vi "Write DAQ Parameters.vi"(8 "error in (no error)":errorcluster, 10 "DAQ Parameters":T1, 11 "ATS9462 Class in":refnum<class "ATS9462 Class.lvclass">) -> (0 "error out":errorcluster, 3 "ATS9462 Class out":refnum<class "ATS9462 Class.lvclass">)   [LabVIEW 2014, in "ATS9462 Class.lvclass"]
uses:
  ATS9462 Class.lvclass
  DAQ Parameters.ctl
  Trigger Source.ctl
  Trigger Slope.ctl
  Type Defs/OCT DAQ Channel Data Type.ctl
  Clock Control.ctl
  ATS-VI/ATS_ctl/ATS_Global.ctl
  ATS-VI/ATS_ctl/Record.ctl
  ATS-VI/ATS_ctl/Clock.ctl
  ATS-VI/ATS_ctl/ClockSource.ctl
  ATS-VI/ATS_ctl/ClockRate.ctl
  ATS-VI/ATS_ctl/ClockEdge.ctl
  ATS-VI/ATS_ctl/InputCtrl.ctl
  ATS-VI/ATS_ctl/Coupling.ctl
  ATS-VI/ATS_ctl/Range.ctl
  ATS-VI/ATS_ctl/Impedance.ctl
  ATS-VI/ATS_ctl/Bandwidth.ctl
  ATS-VI/ATS_ctl/Trigger.ctl
  ATS-VI/ATS_ctl/TriggerOperation.ctl
  ATS-VI/ATS_ctl/TriggerEngine.ctl
  ATS-VI/ATS_ctl/ExtTrigger.ctl
  ATS-VI/ATS_ctl/ExtTrigRange.ctl
  ATS-VI/ATS_ctl/ATS_Async_Ctrl.ctl
  ATS-VI/ATS_ctl/ATS_Async_Mode.ctl
  ATS-VI/ATS_ctl/ATS_ReadSamples.ctl
  ATS-VI/ATS_ctl/ATS_Async_Setting.ctl
  ATS9462 Class.lvclass/ATS9462 Class.ctl
  ATS-VI/ATS_ctl/ATS_DMA_Channel.ctl
  DAQ Class.lvclass
panel:
  out "Return Code":u32
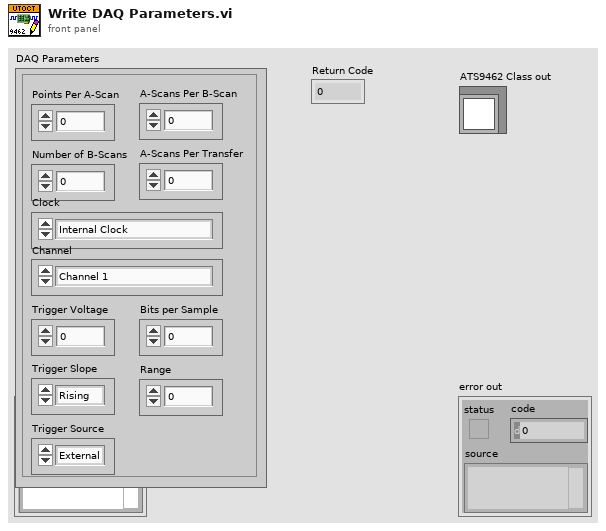
[diagram p1: front panel]
types:
  T1 = typedef "DAQ Class.lvclass/DAQ Parameters.ctl" = cluster{"Points Per A-Scan":u32, "A-Scans Per B-Scan":u32, "Number of B-Scans":u32, "A-Scans Per Transfer":u32, "Trigger Voltage":sgl, "Trigger Source":T2, "Trigger Slope":T3, "Channel":T4, "Clock":T5, "Bits per Sample":dbl, "Range":dbl}
  T2 = typedef "DAQ Class.lvclass/Trigger Source.ctl" = enum16{"External", "Channel A", "Channel B"}
  T3 = typedef "DAQ Class.lvclass/Trigger Slope.ctl" = enum16{"Rising", "Falling"}
  T4 = typedef "OCT DAQ Channel Data Type.ctl" = enum16{"Channel 1", "Channel 2", "Channel 1 and 2"}
  T5 = typedef "DAQ Class.lvclass/Clock Control.ctl" = enum16{"Internal Clock", "External Clock"}
  T6 = typedef "ClockRate.ctl" = u32
  T7 = typedef "ATS_Async_Setting.ctl" = cluster{"UseHeader":u32, "Rec/Buffer":u32, "Total_Rec":u32, "DataBuffer":bool, "GetProcessedData":bool}
  T8 = typedef "ATS_ReadSamples.ctl" = cluster{"Offset":i32, "Length":u32}
  T9 = typedef "ATS_Async_Mode.ctl" = enum16{"Continuous", "Triggered", "No-Pre-Trigger", "Traditional"}
  T10 = typedef "ATS_Async_Ctrl.ctl" = enum16{"SetupDMA", "StartCapture", "Get", "Get_Stream", "Abort", "Stop"}
  T11 = typedef "ATS_Global.ctl" = cluster{"Record":T12, "Clock":T13, "Input A":T16, "Input B":T16, "Trigger":T21}
  T12 = typedef "Record.ctl" = cluster{"Count":u32, "Presize":u32, "Length":u32}
  T13 = typedef "Clock.ctl" = cluster{"ClckSource":T14, "ClckRate":T6, "ClckEdge":T15, "Decimation":u32}
  T14 = typedef "ClockSource.ctl" = enum16{"Internal", "External", "Medium Ext.", "Slow Ext.", "Ext. AC", "Ext. DC", "Ext. (PLL)"}
  T15 = typedef "ClockEdge.ctl" = u16
  T16 = typedef "InputCtrl.ctl" = cluster{"Coupling":T17, "Range":T18, "Impedance":T19, "Bandwidth":T20}
  T17 = typedef "Coupling.ctl" = enum16{"AC", "DC"}
  T18 = typedef "Range.ctl" = u32
  T19 = typedef "Impedance.ctl" = enum16{"1M ohms", "50 ohms"}
  T20 = typedef "Bandwidth.ctl" = enum16{"Full Bandwidth", "Reduce Bandwidth"}
  T21 = typedef "Trigger.ctl" = cluster{"TrigOperation":T22, "Timeout (s)":dbl, "Trig. Delay":u32, "Engine X":T23, "Engine Y":T23, "ExtTrigControl":T24}
  T22 = typedef "TriggerOperation.ctl" = enum16{"Only X", "Only Y", "X or Y", "X and Y", "X xor Y", "X and not Y", "not X and Y"}
  T23 = typedef "TriggerEngine.ctl" = cluster{"Source":enum32{"Chan_A", "Chan_B", "External", "Disable"}, "Slope":enum32{"Positive", "Negative"}, "Level":u32}
  T24 = typedef "ExtTrigger.ctl" = cluster{"Coupling":T17, "Range":T25}
  T25 = typedef "ExtTrigRange.ctl" = enum16{"1 V", "5 V", "TTL"}
  T26 = enum32{"Chan_A", "Chan_B", "External", "Disable"}
  T27 = typedef "ATS_DMA_Channel.ctl" = enum16{"Channel_A", "Channel_B", "A & B"}
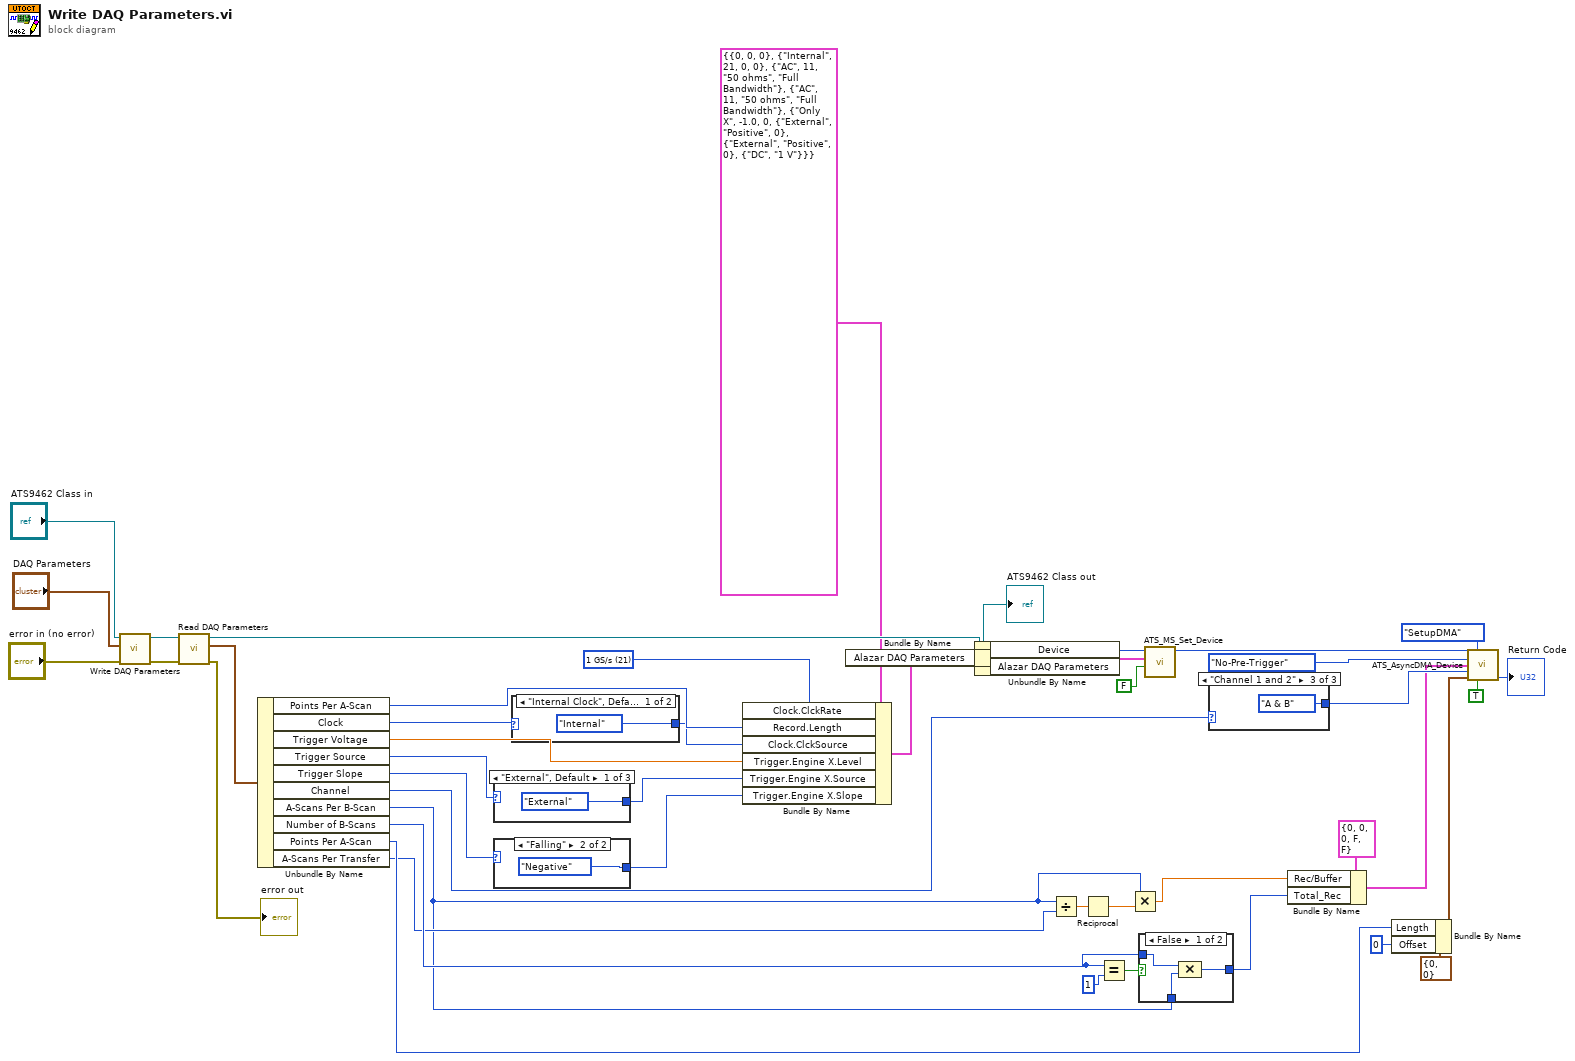
[diagram p0: block diagram]
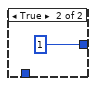
[diagram p2: hidden frame]
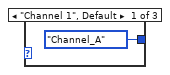
[diagram p3: hidden frame]
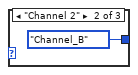
[diagram p4: hidden frame]
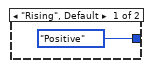
[diagram p5: hidden frame]
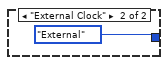
[diagram p6: hidden frame]
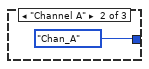
[diagram p7: hidden frame]
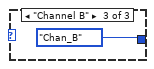
[diagram p8: hidden frame]
diagram:
  w11 = T6 21 items=["1 kS/s", "2 kS/s", "5 kS/s", "10 kS/s", "20 kS/s", "50 kS/s", "100 kS/s", "200 kS/s", "500 kS/s", "1 MS/s", "2 MS/s", "5 MS/s", "10 MS/s", "20 MS/s", "25 MS/s", "50 MS/s", "100 MS/s", "125 MS/s", "200 MS/s", "250 MS/s", "500 MS/s", "1 GS/s"] ("Clock.ClckRate")
  n1 = call-parent "Write DAQ Parameters.vi"("error in (no error)"="error in (no error)", "DAQ Parameters"="DAQ Parameters", "DAQ Class in"="ATS9462 Class in") -> ("error out"=w41:errorcluster, "DAQ Class out"=w42:refnum<class "ATS9462 Class.lvclass">)  [unwired: 7 in]
  n2 = call-dynamic "Read DAQ Parameters.vi"("error in (no error)"=w41, "ATS9462 Class in"=w42) -> ("error out"=→"error out":errorcluster, "DAQ Parameters"=w40:T1, "ATS9462 Class out"=w33:refnum<class "ATS9462 Class.lvclass">)  [unwired: 7 in]
  n3 = Unbundle By Name(w40) -> ("Points Per A-Scan"=w37:u32, "Clock"=w36:T5, "Trigger Voltage"=w34:sgl, "Trigger Source"=w39:T2, "Trigger Slope"=w32:T3, "Channel"=w24:T4, "A-Scans Per B-Scan"=w1:u32, "Number of B-Scans"=w7:u32, "Points Per A-Scan"=w13:u32, "A-Scans Per Transfer"=w2:u32)
  n4 = case shown="\"External\", Default" w39 {
    tunnel: [T26."External" ("Trigger.Engine X.Source") T26."Chan_A" ("Trigger.Engine X.Source") T26."Chan_B" ("Trigger.Engine X.Source")] -> w38
    frame "External", Default {
    }
    frame "Channel A" {
    }
    frame "Channel B" {
    }
  }
  n5 = case shown="\"Falling\"" w32 {
    tunnel: [enum32{"Positive", "Negative"}."Positive" ("Trigger.Engine X.Slope") enum32{"Positive", "Negative"}."Negative" ("Trigger.Engine X.Slope")] -> w31
    frame "Rising", Default {
    }
    frame "Falling" {
    }
  }
  n6 = case shown="\"Internal Clock\", Default" w36 {
    tunnel: [ClockSource."Internal" ("Clock.ClckSource") ClockSource."External" ("Clock.ClckSource")] -> w35
    frame "Internal Clock", Default {
    }
    frame "External Clock" {
    }
  }
  n7 = Bundle By Name(cluster=T11 {"Record"={"Count"=0, "Presize"=0, "Length"=0}, "Clock"={"ClckSource"=enum."Internal", "ClckRate"=21, "ClckEdge"=0, "Decimation"=0}, "Input A"={"Coupling"=enum."AC", "Range"=11, "Impedance"=enum."50 ohms", "Bandwidth"=enum."Full Bandwidth"}, "Input B"={"Coupling"=enum."AC", "Range"=11, "Impedance"=enum."50 ohms", "Bandwidth"=enum."Full Bandwidth"}, "Trigger"={"TrigOperation"=enum."Only X", "Timeout (s)"=-1.0, "Trig. Delay"=0, "Engine X"={"Source"=enum."External", "Slope"=enum."Positive", "Level"=0}, "Engine Y"={"Source"=enum."External", "Slope"=enum."Positive", "Level"=0}, "ExtTrigControl"={"Coupling"=enum."DC", "Range"=enum."1 V"}}} ("Value"), "Clock.ClckRate"=w11, "Record.Length"=w37, "Clock.ClckSource"=w35, "Trigger.Engine X.Level"=w34, "Trigger.Engine X.Source"=w38, "Trigger.Engine X.Slope"=w31) -> (w23:T11)
  n8 = Bundle By Name(cluster=w33, "Alazar DAQ Parameters"=w23) -> (w17:refnum<class "ATS9462 Class.lvclass">)
  "ATS9462 Class out" <- w17
  n9 = Unbundle By Name(w17) -> ("Device"=w21:i32, "Alazar DAQ Parameters"=w20:T11)
  n10 = Divide(x=w1, y=w2) -> (x/y=w5:dbl)
  n11 = Reciprocal(x=w5) -> (1/x=w4:dbl)
  n12 = Equal?(x=w7, y=u32 1) -> (x = y?=w9:bool)
  n13 = Multiply(x=w1, y=w4) -> (x*y=w3:dbl)
  n14 = case shown="False" w9 {
    tunnel: [w55 u32 1 ("y")] -> w8
    tunnel: w7 -> [w54 _]
    tunnel: w1 -> [w53 _]
    frame False {
      n15 = Compound Arithmetic op=MULTIPLY(w54, w53) -> (w55:u32)
    }
    frame True {
    }
  }
  n16 = call "ATS_MS_Set_Device.vi"("Set_Manually (F)"=FALSE, "Setup_In"=w20, "DeviceIn"=w21) -> ("DeviceOut"=w18:i32)  [unwired: 3 in, 5 out]
  n17 = case shown="\"Channel 1 and 2\"" w24 {
    tunnel: [ATS_DMA_Channel."Channel_A" ("Channel") ATS_DMA_Channel."Channel_B" ("Channel") ATS_DMA_Channel."A & B" ("Channel")] -> w30
    frame "Channel 1", Default {
    }
    frame "Channel 2" {
    }
    frame "Channel 1 and 2" {
    }
  }
  n18 = Bundle By Name(cluster=T7 {"UseHeader"=0, "Rec/Buffer"=0, "Total_Rec"=0, "DataBuffer"=FALSE, "GetProcessedData"=FALSE} ("Async_Setting"), "Rec/Buffer"=w3, "Total_Rec"=w8) -> (w15:T7)
  n19 = Bundle By Name(cluster=T8 {"Offset"=0, "Length"=0} ("ReadSamples"), "Length"=w13, "Offset"=0) -> (w28:T8)
  n20 = call "ATS_AsyncDMA_Device.vi"("DeviceIn"=w18, "ATS_Async_Ctrl"=ATS_Async_Ctrl."SetupDMA" ("ATS_DMA_Ctrl"), "Async_Mode"=ATS_Async_Mode."No-Pre-Trigger", "Async_Setting"=w15, "Channel"=w30, "ReadSamples"=w28, "Start Now / Wait"=TRUE) -> ("Return Code"=→"Return Code":u32)  [unwired: 4 in, 4 out]
